vi "launch labview if not running.vi"(8 "error in":errorcluster, 9 "exe path":path, 10 "lv path specified":bool, 11 "desired lv version":dbl) -> (0 "error out":errorcluster, 1 "newly opened":bool, 2 "port":u32, 3 "vi server available":bool, 5 "labview directory":path)   [LabVIEW 2018]
uses:
  <vilib>/Utility/config.llb/Read Key (String).vi
  <vilib>/Utility/config.llb/Read Key (U32).vi
  <vilib>/Utility/config.llb/NI_LVConfig.lvlib
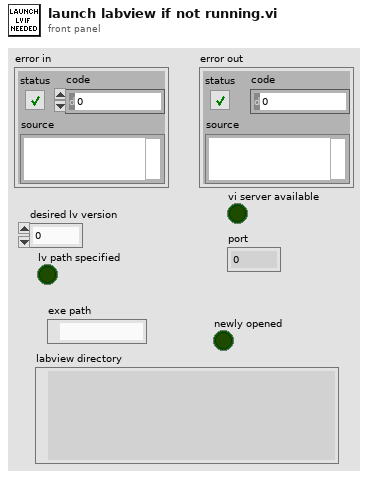
[diagram p1: front panel]
types:
  T1 = typedef "NI_LVConfig.lvlib/Config Data RefNum.ctl" = refnum<k1>
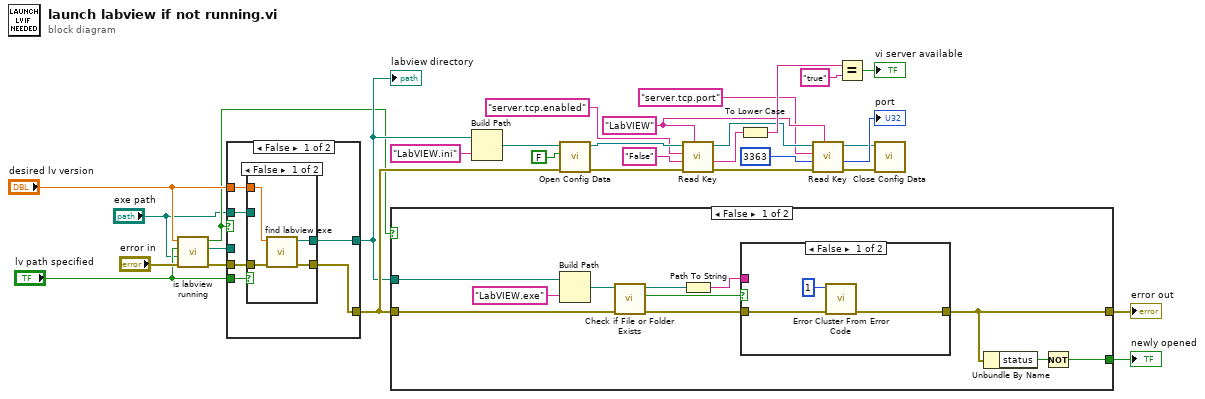
[diagram p0: block diagram]
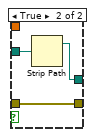
[diagram p2: hidden frame]
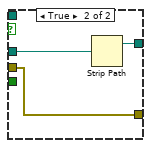
[diagram p3: hidden frame]
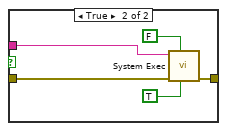
[diagram p4: hidden frame]
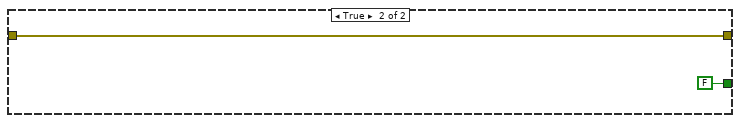
[diagram p5: hidden frame]
diagram:
  w8 = "LabVIEW" ("section")
  n1 = call "is labview running.vi"("error in"="error in", "exe path specified"="exe path", "lv path specified"="lv path specified", "labview version"="desired lv version") -> ("error out"=w29:errorcluster, "exe path"=w3:path, "running"=w4:bool)  [unwired: 5 in]
  n2 = case shown="False" w4 {
    tunnel: w29 -> [w36 w46]
    tunnel: [w35 w46] -> w20
    tunnel: [w34 w44] -> w18
    tunnel: "desired lv version" -> [w33 _]
    tunnel: w3 -> [_ w45]
    tunnel: "lv path specified" -> [w32 _]
    tunnel: "exe path" -> [w31 _]
    frame False {
      n3 = case shown="False" w32 {
        tunnel: w36 -> [w40 w43]
        tunnel: [w39 w43] -> w35
        tunnel: [w38 w41] -> w34
        tunnel: w33 -> [w37 _]
        tunnel: w31 -> [_ w42]
        frame False {
          n4 = call "find labview exe.vi"("error in"=w40, "desired lv version"=w37) -> ("error out"=w39:errorcluster, "labview directory"=w38:path)  [unwired: 8 in]
        }
        frame True {
          n5 = Strip Path(path=w42) -> (stripped path=w41:path)  [unwired: 1 out]
        }
      }
    }
    frame True {
      n6 = Strip Path(path=w45) -> (stripped path=w44:path)  [unwired: 1 out]
    }
  }
  "labview directory" <- w18
  n7 = case shown="False" w4 {
    tunnel: [w50 w67] -> w21
    tunnel: w20 -> [w48 w67]
    tunnel: [w49 FALSE] -> w19
    tunnel: w18 -> [w47 _]
    frame False {
      n8 = Build Path(base path=w47, name or relative path="LabVIEW.exe") -> (appended path=w51:path)
      n9 = call <vilib>:"Check if File or Folder Exists.vi"("error in (no error)"=w48, "path"=w51) -> ("error out"=w56:errorcluster, "file or folder exists?"=w57:bool, "dup path"=w55:path)  [unwired: 7 in]
      n10 = Path To String(path=w55) -> (string=w54:string)
      n11 = case shown="False" w57 {
        tunnel: [w59 w64] -> w50
        tunnel: w56 -> [w60 w65]
        tunnel: w54 -> [_ w63]
        frame False {
          n12 = call <vilib>:"Error Cluster From Error Code.vi"("error in (no error)"=w60, "error code (0)"=1) -> ("error out"=w59:errorcluster)  [unwired: 7 in]
        }
        frame True {
          n13 = call <vilib>:"System Exec.vi"("run minimized? (F)"=TRUE, "wait until completion? (T)"=FALSE, "error in (no error)"=w65, "command line"=w63) -> ("error out"=w64:errorcluster)  [unwired: 4 in, 3 out]
        }
      }
      n14 = Unbundle By Name(w50) -> ("status"=w53:bool)
      n15 = Not(x=w53) -> (.not. x?=w49:bool)
    }
    frame True {
    }
  }
  "error out" <- w21
  "newly opened" <- w19
  n16 = Build Path(base path=w18, name or relative path="LabVIEW.ini") -> (appended path=w23:path)
  n17 = call <vilib>:"Open Config Data.vi"("error in (no error)"=w20, "create file if necessary (T)"=FALSE, "configuration file path"=w23) -> ("error out"=w12:errorcluster, "refnum"=w13:T1)  [unwired: 6 in, 1 out]
  n18 = call-poly <vilib>:"Read Key.vi"("section"=w8, "error in (no error)"=w12, "default value"="False", "key"="server.tcp.enabled", "refnum"=w13) -> ("error out"=w14:errorcluster, "value"=w22:string, "refnum out"=w15:T1)  [unwired: 3 in, 1 out]
  n19 = To Lower Case(string=w22) -> (all lower case string=w26:string)
  n20 = call-poly <vilib>:"Read Key.vi"("section"=w8, "error in (no error)"=w14, "default value"=u32 3363, "key"="server.tcp.port", "refnum"=w15) -> ("error out"=w17:errorcluster, "value"=→"port":u32, "refnum out"=w16:T1)  [unwired: 3 in, 1 out]
  n21 = Equal?(x=w26, y="true") -> (x = y?=→"vi server available":bool)
  n22 = call <vilib>:"Close Config Data.vi"("error in (no error)"=w17, "refnum"=w16) -> ()  [unwired: 8 in, 2 out]
